vi "ModbusSlave.vi"() -> ()   [LabVIEW 2020]
uses:
  <vilib>/NI/Modbus Library/API/Wrapper/Create TCP Slave.vi
  <vilib>/NI/Modbus Library/API/Slave/Modbus Slave.lvclass
  <vilib>/NI/Modbus Library/API/Wrapper/API Main.lvlib
panel:
  in  "stop":bool
  out "Coils":bool[](array[boolean])
  out "Array":u16[](array[slide]) scale=0.0..100.0
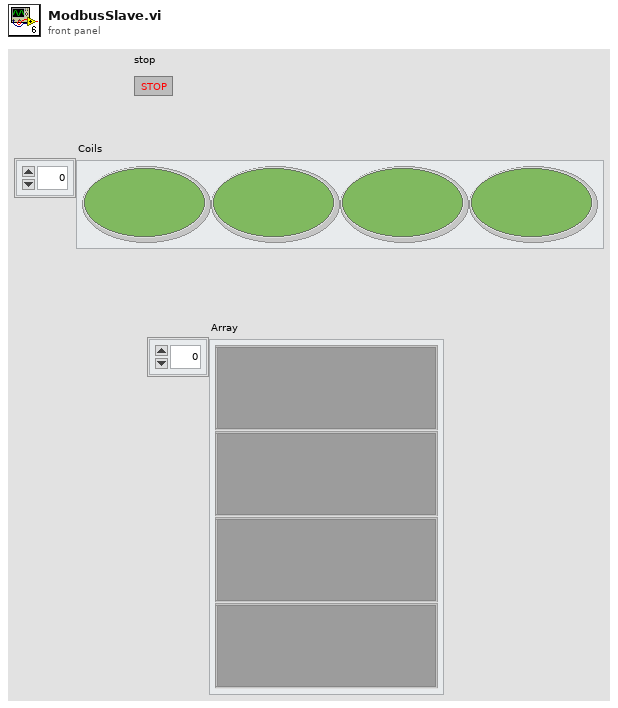
[diagram p1: front panel]
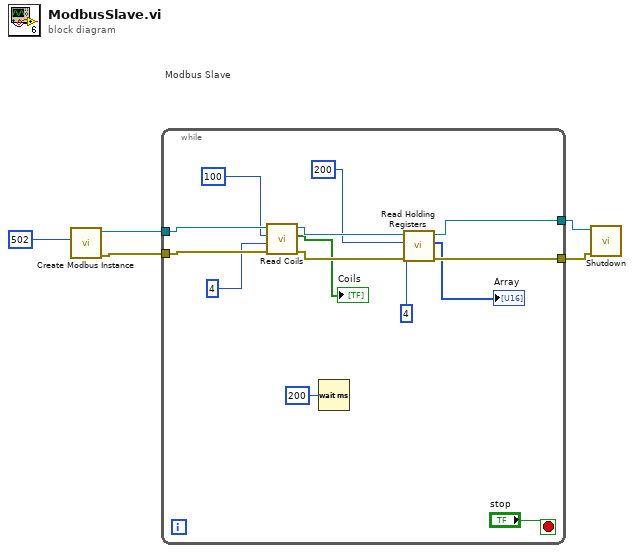
[diagram p0: block diagram]
diagram:
  # "Modbus Slave"
  n1 = call-poly <vilib>:"Create Modbus Instance.vi"("port (502)"=u16 502) -> ("error out"=w3:errorcluster, "TCP slave instance"=w4:refnum<class "Modbus Slave.lvclass">)  [unwired: 9 in]
  n2 = while {
    tunnel: w4 -> [w17]
    tunnel: w3 -> [w12]
    tunnel: [w15] -> w2
    tunnel: [w14] -> w1
    stop <- "stop" stop-if-true
    n3 = call-dynamic "Read Coils.vi"("error in"=w12, "number of inputs"=u16 4, "starting address"=u16 100, "Modbus slave in"=w17) -> ("error out"=w13:errorcluster, "coils"=→"Coils":bool[], "Modbus slave out"=w16:refnum<class "Modbus Slave.lvclass">)  [unwired: 5 in]
    n4 = Wait (ms)(milliseconds to wait=u32 200) -> ()  [unwired: 1 out]
    n5 = call-dynamic "Read Holding Registers.vi"("error in"=w13, "number of inputs"=u16 4, "starting address"=u16 200, "Modbus slave in"=w16) -> ("error out"=w14:errorcluster, "register values"=→"Array":u16[], "Modbus slave out"=w15:refnum<class "Modbus Slave.lvclass">)  [unwired: 5 in]
  }
  n6 = call-dynamic "Shutdown.vi"("error in"=w1, "Modbus slave in"=w2) -> ()  [unwired: 9 in, 1 out]
